vi "ReportADCResultsInVoltsTSFTS2.vi"(6 "Blue Board Enum":T1=enum."INVB_UDC", 7 "Green Board Enum":T3, 8 "error in (no error)":errorcluster, 9 "Message IN":string, 10 "Board Selector":T2) -> (0 "error out":errorcluster, 1 "Message OUT":string, 2 "Result":dbl, 3 "VISA Refnum out":refnum<visa-resource-name>)   [LabVIEW 2022 SP3]
uses:
  ADCSelector GB.ctl
  Board Select.ctl
  ADCSelector BB.ctl
  <vilib>/Instr/_visa.llb/VISA Flush IO Buffer Mask.ctl
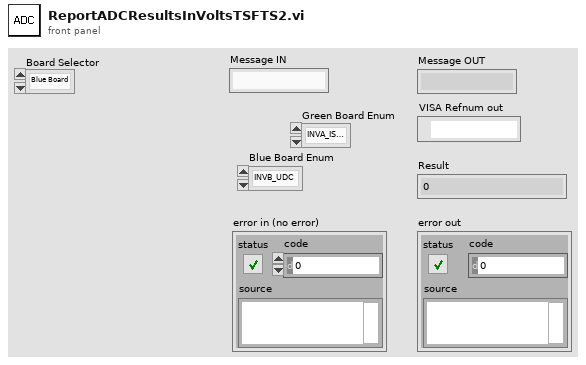
[diagram p1: front panel]
types:
  T1 = typedef "ADCSelector BB.ctl" = enum16{"INVA_ISENSE_U", "INVA_ISENSE_V", "INVA_ISENSE_W", "INVA_UDC", "INVA_TEMP", "HB_TEMP", "AUXB_TEMP", "VLINE_AB", "VLINE_BC", "VLINE_CA", "VSENSE_POS_24V", "VSENSE_POS_5V", "VSENSE_NEG_15V", "INVB_ISENSE_U", "INV_B_ISENSEV", "INVB_ISENSE_W", "INVB_UDC", "INVB_TEMP", "AUXA_TEMP", "AUXC_TEMP", "VOUT_AB", "VOUT_BC", "VOUT_CA", "VSENSE_POS_15V", "VSENSE_POS_3P3V", "TEST_POINT"}
  T2 = typedef "Board Select.ctl" = enum16{"Blue Board", "Green Board"}
  T3 = typedef "ADCSelector GB.ctl" = enum16{"INVA_ISENSE_U", "INVA_ISENSE_V", "INVA_ISENSE_W", "INVA_UDC", "INVA_TEMP", "HB_ISENSE", "AUX_ISENSE_U", "AUX_ISENSE_V", "AUX_ISENSE_W", "VLINE_AB", "VLINE_BC", "VLINE_CA", "REF_1P5V", "VSENSE_POS_24V", "VSENSE_POS_5V", "VSENSE_NEG_15V", "TEST_POINT", "INVB_ISENSE_U", "INVB_ISENSE_V", "INVB_ISENSE_W", "INVB_UDC", "INVB_TEMP", "HB_TEMP", "AUXA_TEMP", "AUXB_TEMP", "AUXC_TEMP", "VOUT_AB", "VOUT_BC", "VOUT_CA", "REF_2P5V", "VSENSE_POS_15V", "VSENSE_POS_3P3V", "NET_ANALYZER"}
  T4 = typedef "VISA Flush IO Buffer Mask.ctl" = u16
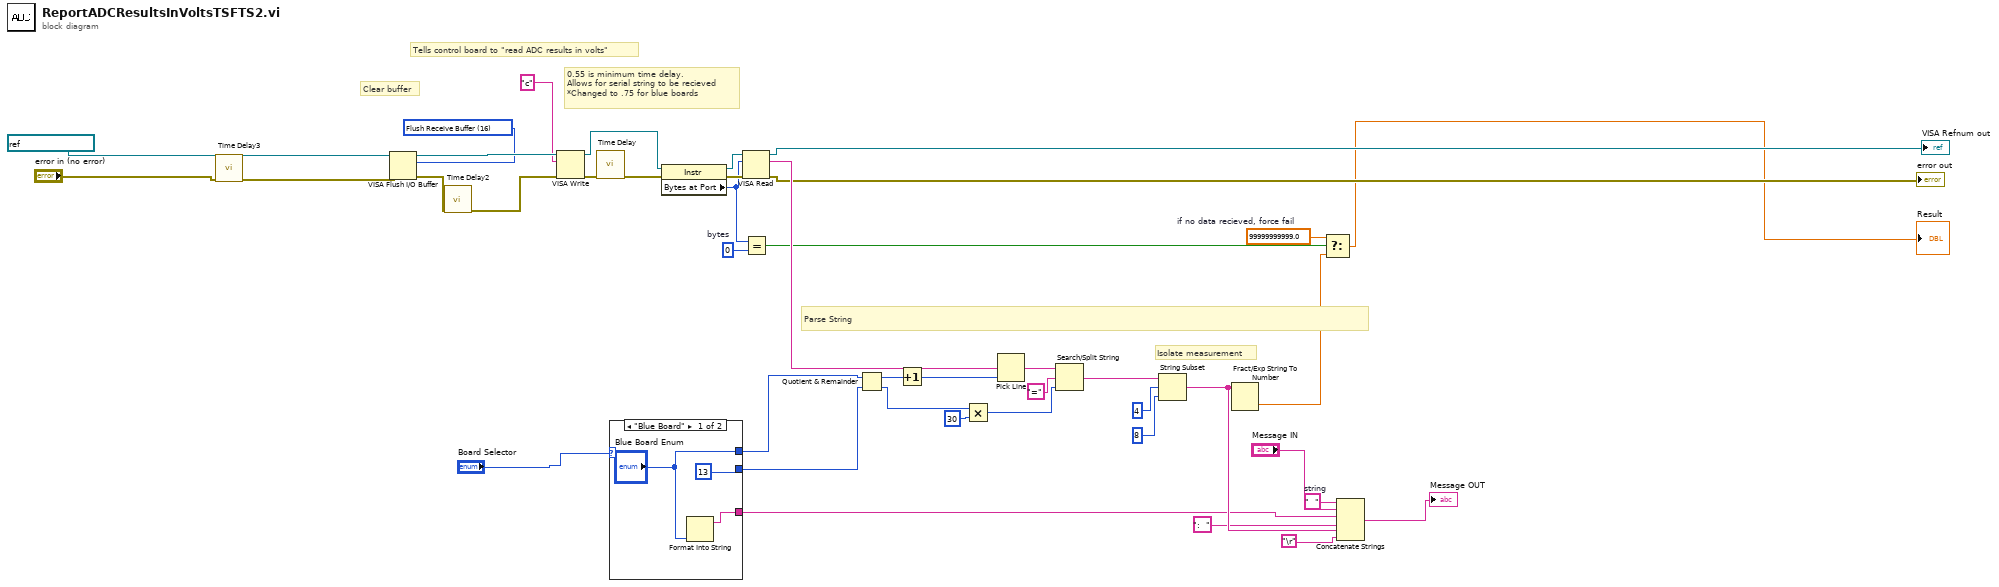
[diagram p0: block diagram]
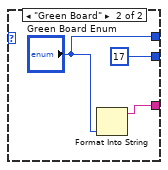
[diagram p2: hidden frame]
diagram:
  w13 = "  "  # string
  w19 = 99999999999.0  # if no data recieved, force fail
  w22 = u32 0  # bytes
  w27 = T4 16 items=["Flush Receive Buffer"=16, "Write Transmit Buffer to Device"=32, "Flush Receive Buffer (No I/O)"=64, "Flush Transmit Buffer"=128] ("Mask")
  # "Isolate measurement"
  # "Clear buffer"
  # "Parse String"
  # "0.55 is minimum time delay.\nAllows for serial string to be recieved\n*Changed to .75 for blue boards"
  # "Tells control board to \"read ADC results in volts\""
  n1 = call "Time Delay3"("error in (no error)"="error in (no error)") -> ("error out"=w1:errorcluster)  [unwired: 10 in]
  n2 = VISA Flush I/O Buffer(VISA resource name=refnum<visa-resource-name> "ControlBoard" ("VISA Refnum in"), mask (16)=w27, error in (no error)=w1) -> (VISA resource name out=w29:refnum<visa-resource-name>, error out=w4:errorcluster)
  n3 = call "Time Delay2"("error in (no error)"=w4) -> ("error out"=w3:errorcluster)  [unwired: 10 in]
  n4 = VISA Write(VISA resource name=w29, write buffer="c", error in (no error)=w3) -> (VISA resource name out=w31:refnum<visa-resource-name>, error out=w28:errorcluster)  [unwired: 1 out]
  n5 = call "Time Delay"("error in (no error)"=w28) -> ("error out"=w30:errorcluster)  [unwired: 10 in]
  n6 = case shown="\"Blue Board\"" "Board Selector" {
    tunnel: ["Blue Board Enum" "Green Board Enum"] -> w8
    tunnel: [13 17] -> w7
    tunnel: [w44 w46] -> w6
    frame "Blue Board" {
      n7 = Format Into String("Blue Board Enum") -> (resulting string=w44:string)  [unwired: 3 in, 1 out]
    }
    frame "Green Board" {
      n8 = Format Into String("Green Board Enum") -> (resulting string=w46:string)  [unwired: 3 in, 1 out]
    }
  }
  n9 = property class="Instr"(reference=w31, error in=w30) -> (reference out=w25:refnum<visa-resource-name>, error out=w26:errorcluster, "Bytes at Port"=w23:u32)
  n10 = VISA Read(VISA resource name=w25, byte count=w23, error in (no error)=w26) -> (VISA resource name out=→"VISA Refnum out":refnum<visa-resource-name>, read buffer=w40:string, error out=→"error out":errorcluster)  [unwired: 1 out]
  n11 = Equal?(x=w23, y=w22) -> (x = y?=w20:bool)
  n12 = Quotient & Remainder(x=w8, y=w7) -> (x-y*floor(x/y)=w35:i32, floor(x/y)=w37:i32)
  n13 = Increment(x=w35) -> (x+1=w36:i32)
  n14 = Multiply(x=w37, y=30) -> (x*y=w39:i32)
  n15 = Pick Line(multi-line string=w40, line index=w36) -> (output string=w41:string)  [unwired: 1 in]
  n16 = Search/Split String(string=w41, search string/char (-)="=" ("regular expression"), offset (0)=w39) -> (match + rest of string=w33:string)  [unwired: 2 out]
  n17 = String Subset(string=w33, offset (0)=4, length (rest)=8 ("offset (0)")) -> (substring=w15:string)
  n18 = Fract/Exp String To Number(string=w15) -> (number=w21:dbl)  [unwired: 3 in, 1 out]
  n19 = Select(t=w19, s=w20, f=w21) -> (s? t:f=→"Result":dbl)
  n20 = Concatenate Strings(w13, "Message IN", w6, ":  ", w15, "\r") -> (→"Message OUT":string)
